vi "DCSAnalysis.vi"(0 "# Detectors":u32=8, 2 "File path":string, 3 "Frame #":u32, 5 "rho":dbl[](array[numeric])=[2.5, 2.5, 2.5, 2.5, 2.5, 2.5, 2.5, 2.5, -1.0, -1.0, -1.0, -1.0], 7 "other settings":u32[](array[numeric])=[0, 0, 0, 0, 0, 0, 0, 0, 0, 0, 0, 0], 8 "avgBool":bool[][](array[boolean]), 9 "var values":dbl[](array[numeric])=[0.0, 0.0, 0.0, 0.0, -1.0, -1.0, -1.0, -1.0, -1.0, -1.0, -1.0, -1.0]) -> (20 "Flow in each detector":dbl[](array[numeric])=[-1.0, -1.0, -1.0, -1.0, -1.0, -1.0, -1.0, -1.0, -1.0, -1.0, -1.0, -1.0], 23 "Tau":T1(graph) caption="Relative changes of flow", 26 "error out":errorcluster, 27 "End":bool)   [LabVIEW 2016]
panel:
  in  "Get Flow Function Path":path=path "C:/Users/BUCKLEY-ADMIN/Desktop/DCScode_Penn_Mar2015/DCS&ISS_ERIN/dll.dll"
  out "avgInt1x32":u32[](array[numeric])
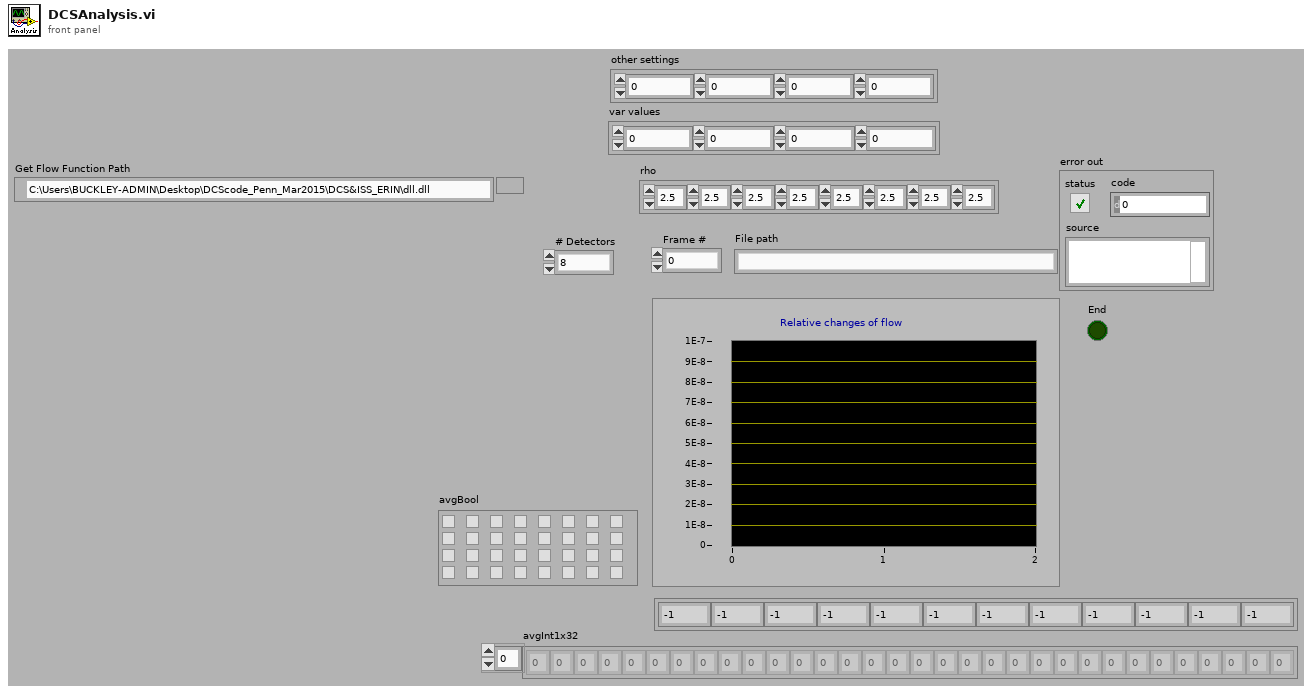
[diagram p1: front panel]
types:
  T1 = cluster{dbl, dbl, dbl, dbl, dbl, dbl, dbl, dbl, dbl, dbl, dbl, dbl}
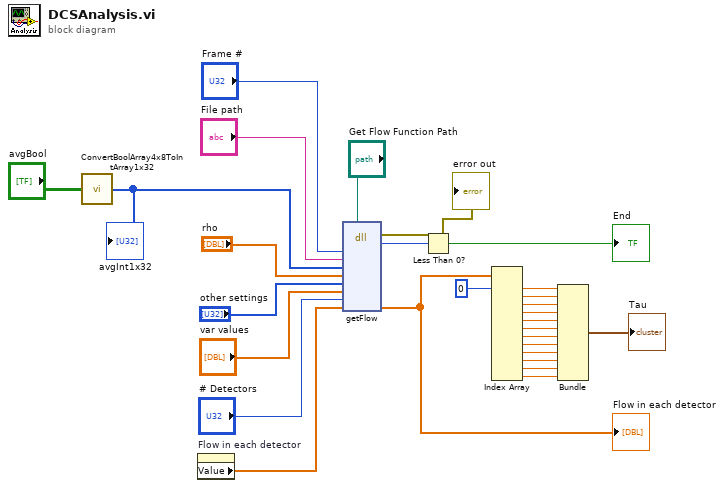
[diagram p0: block diagram]
diagram:
  n1 = call "ConvertBoolArray4x8ToIntArray1x32.vi"("boolMatrix4x8"="avgBool") -> ("intArray1x32"=w28:u32[])  [unwired: 14 in]
  "avgInt1x32" <- w28
  n2 = property on="Flow in each detector" class="Arr (strict)"() -> ("Value"=w22:dbl[])  [unwired: 2 in, 2 out]
  n3 = dll-call lib="C:/Users/BUCKLEY-ADMIN/Desktop/DCScode_Penn_Mar2015/DCS&ISS_ERIN/dll.dll" fn="getFlow"(path in="Get Flow Function Path", "iFileIndex"="Frame #", "fileName"="File path", "avg"=w28, "rho"="rho", "set"="other settings", "var"="var values", "iDetectorCount"="# Detectors", "flow"=w22) -> (error out=→"error out":errorcluster, "return type"=w21:i32, "flow"=w25:dbl[])  [unwired: 9 in, 1 out]
  "Flow in each detector" <- w25
  n4 = Less Than 0?(x=w21) -> (x < 0?=→"End":bool)
  n5 = Index Array(array=w25, index #1=0) -> (element #1=w20:dbl, element #2=w19:dbl, element #3=w18:dbl, element #4=w17:dbl, element #5=w16:dbl, element #6=w15:dbl, element #7=w14:dbl, element #8=w13:dbl, element #9=w10:dbl, element #10=w9:dbl, element #11=w8:dbl, element #12=w7:dbl)  [unwired: 11 in]
  n6 = Bundle(w20, w19, w18, w17, w16, w15, w14, w13, w10, w9, w8, w7) -> (→"Tau":T1)  [unwired: 1 in]
